vi "Destroy.vi"(8 "error in (no error)":errorcluster, 11 "ConfigManager.Cache in":refnum<class "ConfigManager.Cache.lvclass">) -> (0 "error out":errorcluster, 3 "ConfigManager.Cache out":refnum<class "ConfigManager.Cache.lvclass">)   [LabVIEW 2013, in "SMOConfig.lvlib" / "ConfigManager.Cache.lvclass"]
uses:
  ConfigManager.Cache.lvclass
  Manager/ConfigManager.lvclass
  ConfigManager.Cache.lvclass/ConfigManager.Cache.ctl
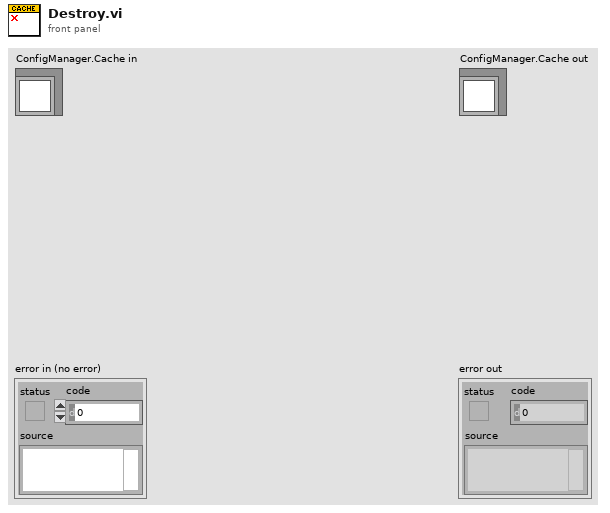
[diagram p1: front panel]
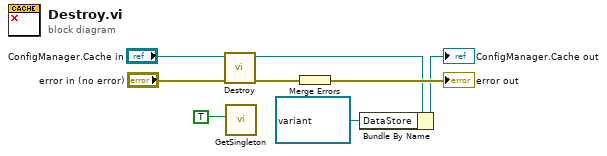
[diagram p0: block diagram]
diagram:
  n1 = call-parent "Destroy.vi"("error in (no error)"="error in (no error)", "ConfigManager in"="ConfigManager.Cache in") -> ("error out"=w6:errorcluster, "ConfigManager out"=w3:refnum<class "ConfigManager.Cache.lvclass">)  [unwired: 8 in]
  n2 = call "GetSingleton.vi"("Destructor (F)"=TRUE ("Creator (F)")) -> ()  [unwired: 9 in, 2 out]
  n3 = Merge Errors(w6) -> (→"error out":errorcluster)
  n4 = Bundle By Name(cluster=w3, "DataStore"=refnum<data-value> refnum) -> (→"ConfigManager.Cache out":refnum<class "ConfigManager.Cache.lvclass">)
